vi "Single Init.vi"(9 "Left Cell Strings":string[](array[string]), 10 "Tree Ref":refnum<vi>) -> ()   [LabVIEW 2025, in "_Shared.lvlib" / "Tree.lvlib"]
uses:
  Tree.lvlib
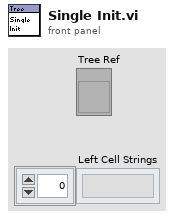
[diagram p1: front panel]
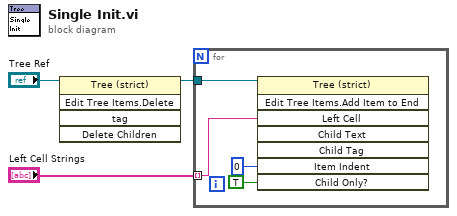
[diagram p0: block diagram]
diagram:
  n1 = invoke class="Tree (strict)" method="Edit Tree Items.Delete"(reference="Tree Ref") -> (reference out=w2:refnum<vi>)  [unwired: 4 in, 4 out]
  n2 = for {
    tunnel: "Left Cell Strings" -> [w4] mode=indexing
    tunnel: w2 -> [w7]
    n3 = invoke class="Tree (strict)" method="Edit Tree Items.Add Item to End"(reference=w7, "Left Cell"=w4, "Item Indent"=0 ("New Item Indentation"), "Child Only?"=TRUE) -> ()  [unwired: 4 in, 8 out]
  }
